vi "Initialize Weather Station.vi"(8 "error in (no error)":errorcluster) -> (0 "error out":errorcluster, 3 "file refnum":refnum<file>, 5 "Weather Data":T1)   [LabVIEW 2010]
doc: "This VI is a part of the Weather Station project. The weather data cluster is created, and a text file (Weather.txt) is created. A header representing the weather data cluster is written to the file.\n\nInputs: Error In\nOutputs: File Refnum, Weather Data Cluster, Error Out"
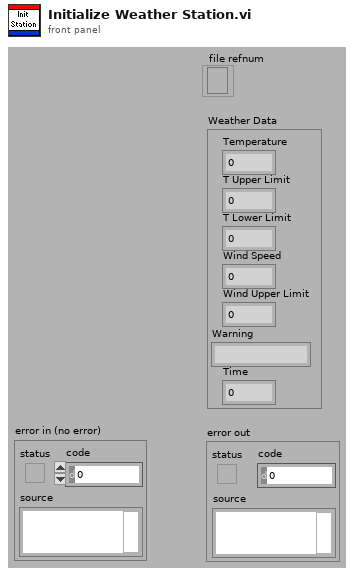
[diagram p1: front panel]
types:
  T1 = cluster{"Temperature":dbl, "T Upper Limit":dbl, "T Lower Limit":dbl, "Wind Speed":dbl, "Wind Upper Limit":dbl, "Warning":string, "Time":dbl}
  T2 = enum16{"open", "replace", "create", "open or create", "replace or create", "replace or create with confirmation"}
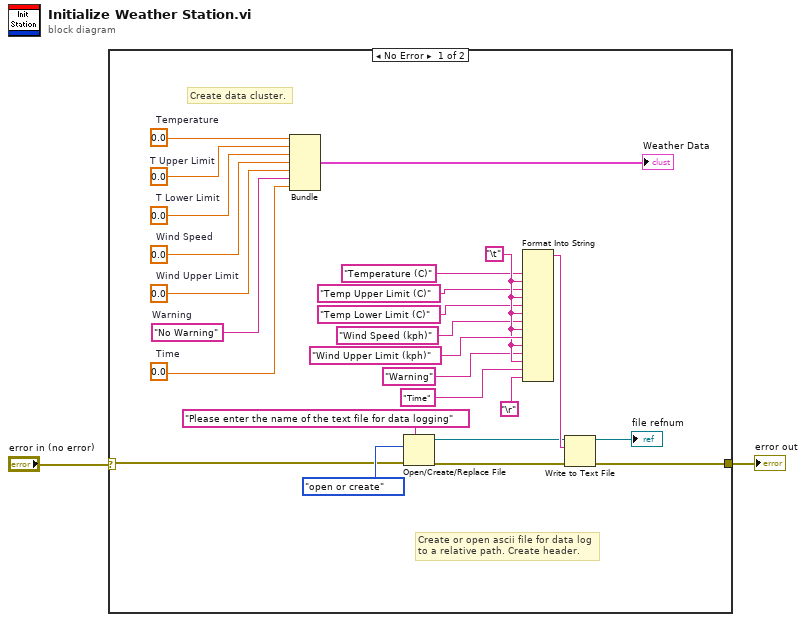
[diagram p0: block diagram]
diagram:
  n1 = case shown="No Error" "error in (no error)" {
    selector: "error in (no error)" -> [w4 w28]
    tunnel: [w26 w28] -> w2
    frame No Error {
      w12 = 0.0  # Time
      w11 = 0.0  # Wind Upper Limit
      w10 = 0.0  # Wind Speed
      w5 = 0.0  # T Lower Limit
      w6 = 0.0  # T Upper Limit
      w7 = 0.0  # Temperature
      w20 = "\t"
      w9 = "No Warning"  # Warning
      # "Create or open ascii file for data log to a relative path. Create header."
      # "Create data cluster."
      n2 = Bundle("Temperature"=w7, "T Upper Limit"=w6, "T Lower Limit"=w5, "Wind Speed"=w10, "Wind Upper Limit"=w11, "Warning"=w9, "Time"=w12) -> (→"Weather Data":T1)  [unwired: 1 in]
      n3 = Open/Create/Replace File(error in=w4, prompt="Please enter the name of the text file for data logging", operation (0:open)=T2."open or create") -> (refnum out=w23:refnum<file>, error out=w25:errorcluster)  [unwired: 3 in, 1 out]
      n4 = Format Into String("Temperature (C)", w20, "Temp Upper Limit (C)", w20, "Temp Lower Limit (C)", w20, "Wind Speed (kph)", w20, "Wind Upper Limit (kph)", w20, "Warning", w20, "Time", "\r") -> (resulting string=w27:string)  [unwired: 3 in, 1 out]
      n5 = Write to Text File(file (use dialog)=w23, text=w27, error in=w25) -> (refnum out=→"file refnum":refnum<file>, error out=w26:errorcluster)  [unwired: 1 in, 1 out]
    }
    frame Error {
    }
  }
  "error out" <- w2
